vi "Power amplifier test.vi"() -> ()   [LabVIEW 2020]
uses:
  FunctionVi/Window/Control/Channel.ctl
  FunctionVi/Queue/Control/QueueState.ctl
  FunctionVi/Window/Control/Bit rate.ctl
  FunctionVi/Window/Control/HwType.ctl
  FunctionVi/Window/Control/Mode.ctl
  <vilib>/Utility/xml.llb/Read From XML File(string).vi
  <vilib>/Utility/file.llb/Write Delimited Spreadsheet (string).vi
  <vilib>/Utility/xml.llb/Read From XML File(array).vi
  <vilib>/Utility/xml.llb/Write to XML File(string).vi
  <userlib>/FTLDCPower/MPD.lvlib
  <userlib>/PCAN-Basic/PCANBasic.lvlib
  FunctionVi/Window/Win_PowerAmplifier_Transmit.vi
panel:
  out "x-y":u32
  out "Status":bool
  out "Company:":string
  out "Time:":string
  out "Channel:":T1 items=["PCAN_USBBUS1"=81, "PCAN_USBBUS2"=82, "PCAN_USBBUS3"=83, "PCAN_USBBUS4"=84]
  in  "PCAN Read error":string
  in  "source":string
  out "Status:":string
  out "Interface Information:":string
  in  "Max voltage:":dbl=30.0 min=5.0 format="%#.3gV"
  in  "BufferTime(s)":dbl=4.0 caption="Buffer:" format="%#.3gs"
  in  "ExecuteTime(s)":dbl=5.0 caption="Execute:" min=1.0 format="%#.3gs"
  in  "Step voltage:":dbl=0.1 format="%#.3gV"
  in  "Max voltage":dbl
  in  "At voltage":dbl
  in  "List record":i32(listbox)
  in  "Reset":bool
  in  "指示灯":bool
  in  "On/Off":bool
  in  "OCPEnable":bool
  in  "OCP:":dbl format="%#.3gA"
  in  "OVPEnable":bool
  in  "OVP:":dbl format="%#.3gV"
  in  "Current:":dbl format="%#.3gA"
  in  "Voltage:":dbl format="%#.3gV"
  in  "Transmit info":bool
  in  "Receive":i32(listbox)
  out "LastError":string
  in  "PCAN Config":bool
  out "Measure Voltage":dbl format="%#.3gV"
  out "Measure Power":dbl format="%#.3gW"
  out "Measure Current":dbl format="%#.3gA"
  in  "RS232 Config":bool
  # "Time"
  # "Output"
  # "Params Set"
  # "Measurement"
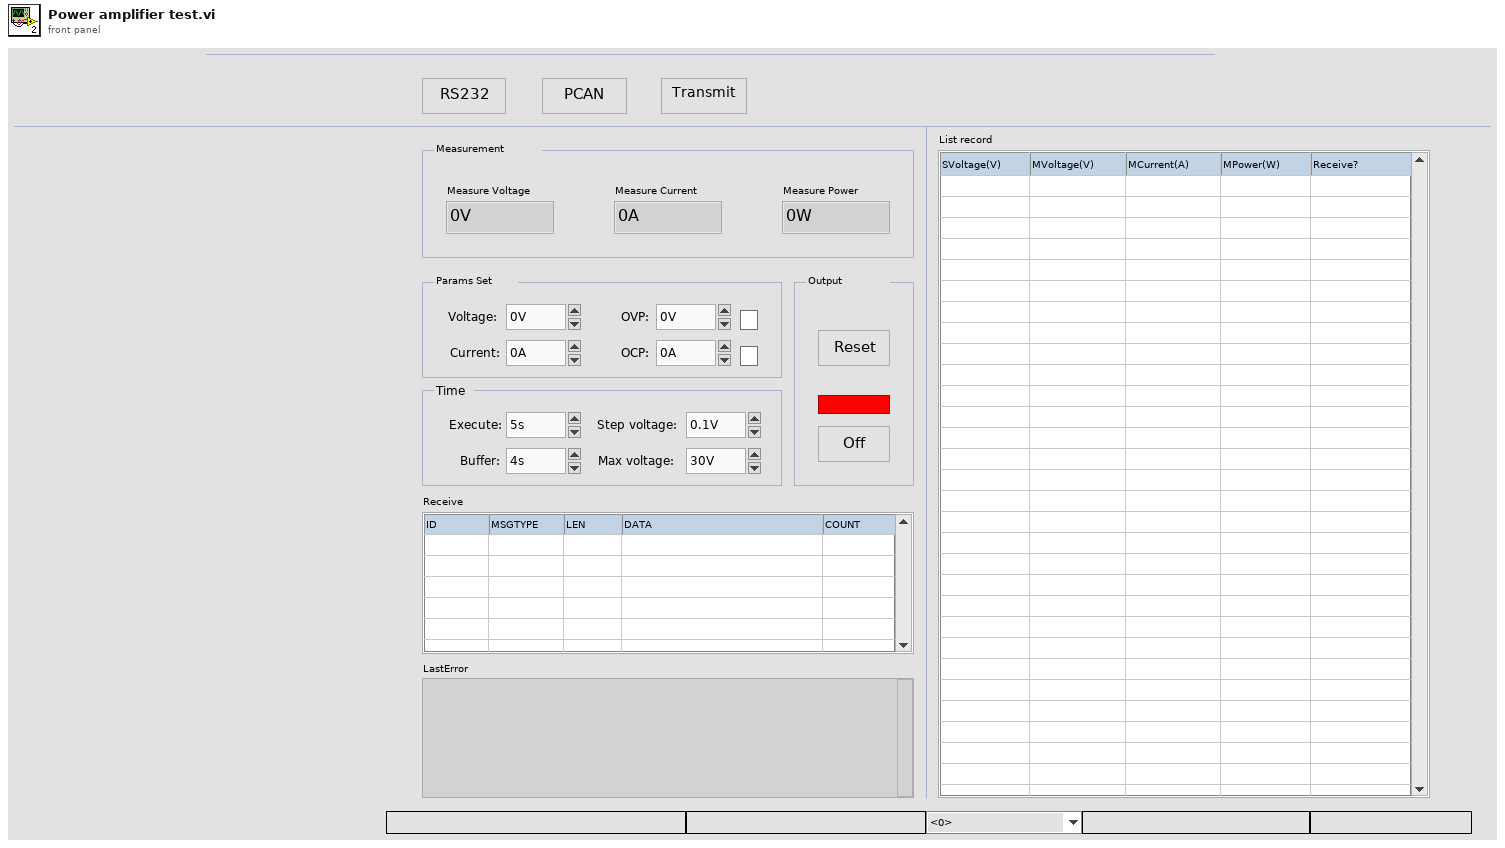
[diagram p1: front panel]
types:
  T1 = typedef "Channel.ctl" = u16
  T2 = typedef "QueueState.ctl" = enum16{"", "Create", "In", "Out", "Empty", "Close"}
  T3 = cluster{"ID":u32, "MSGTYPE":u8, "LEN":u8, "DATA[0]":u8, "DATA[1]":u8, "DATA[2]":u8, "DATA[3]":u8, "DATA[4]":u8, "DATA[5]":u8, "DATA[6]":u8, "DATA[7]":u8}
  T4 = cluster{"Baud Rate":u32, "Parity":u16, "Data Bits":u16, "Stop Bits":u16, "Flow Control":u16}
  T5 = typedef "Mode.ctl" = u8
  T6 = typedef "Bit rate.ctl" = u16
  T7 = typedef "HwType.ctl" = u8
  T8 = enum16{"VOLTage", "DEFault", "MINimum", "MAXimum"}
  T9 = enum16{"current", "DEFault", "MINimum", "MAXimum"}
  T10 = enum8{"Enabled", "Disabled", "Disabled and Grayed Out"}
  T11 = typedef "LVPoint32TypeDef.ctl" = cluster{"Horizontal":i32, "Vertical":i32}
  T12 = typedef "LVRowAndColumnTypeDef.ctl" = cluster{"Row":i32, "Column":i32}
  T13 = cluster{"ID":u32, "MSGTYPE":u8, "LEN":u8, "DATA[0]":u8, "DATA[1]":u8, "DATA[2]":u8, "DATA[3]":u8, "DATA[4]":u8, "DATA[5]":u8, "DATA[6]":u8, "DATA[7]":u8}[]
  T14 = cluster{"Time":u16, "MessageBuffer":cluster{"ID":u32, "MSGTYPE":u8, "LEN":u8, "DATA[0]":u8, "DATA[1]":u8, "DATA[2]":u8, "DATA[3]":u8, "DATA[4]":u8, "DATA[5]":u8, "DATA[6]":u8, "DATA[7]":u8}[]}[]
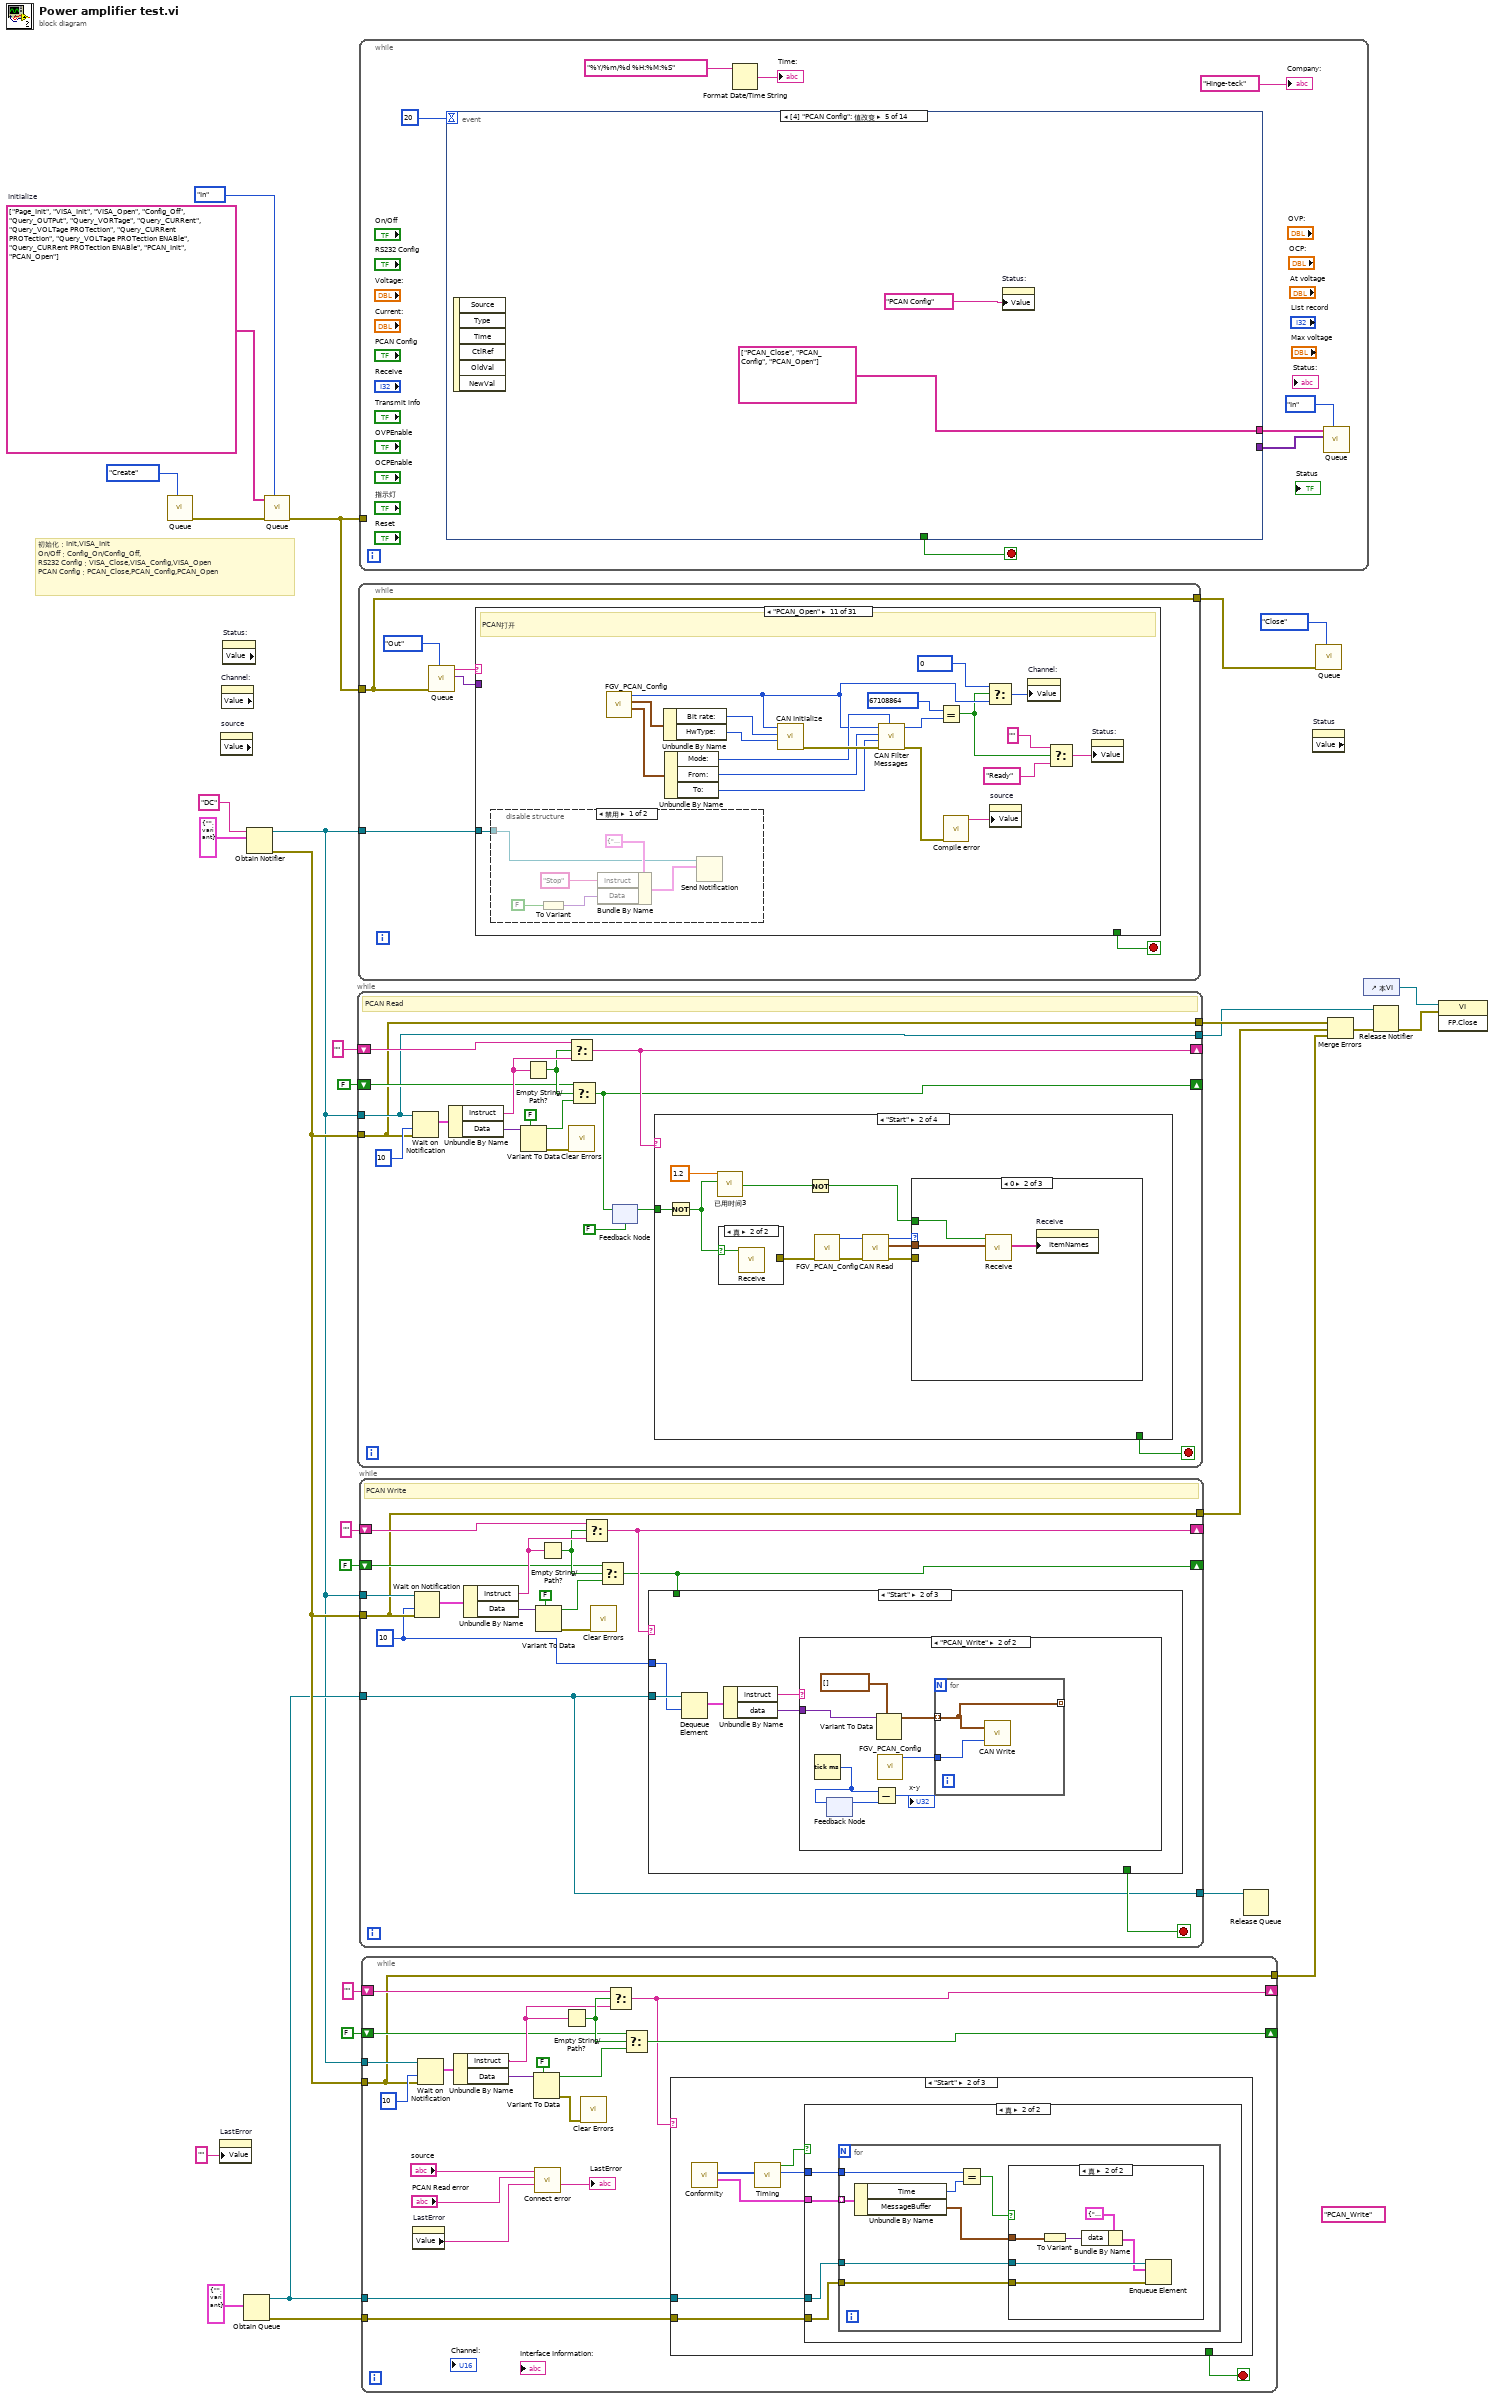
[diagram p0: block diagram]
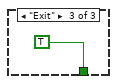
[diagram p5: hidden frame]
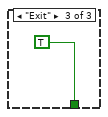
[diagram p8: hidden frame]
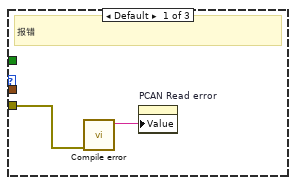
[diagram p10: hidden frame]
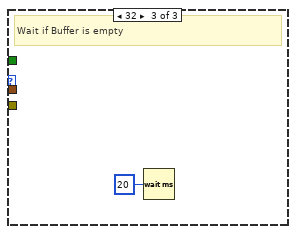
[diagram p11: hidden frame]
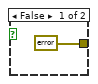
[diagram p12: hidden frame]
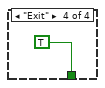
[diagram p14: hidden frame]
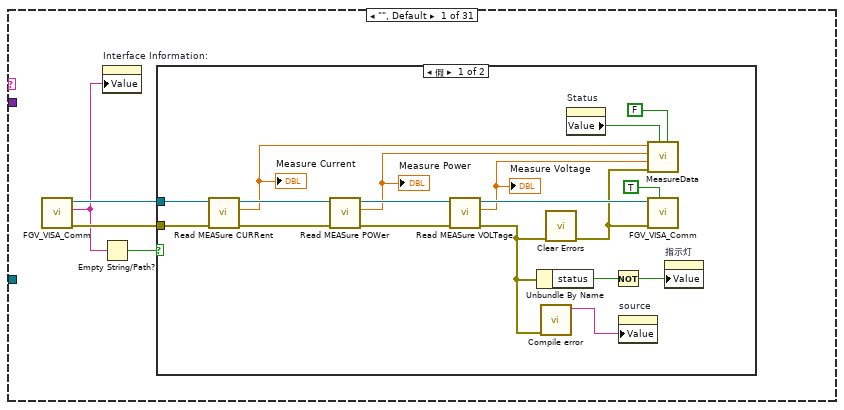
[diagram p15: hidden frame]
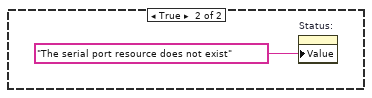
[diagram p16: hidden frame]
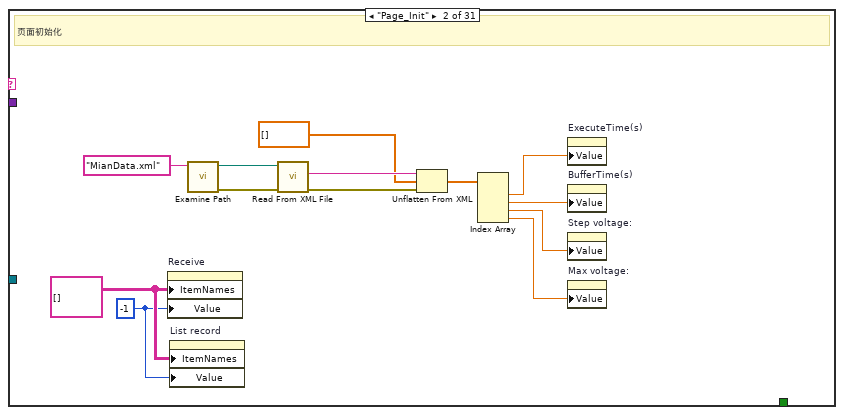
[diagram p17: hidden frame]
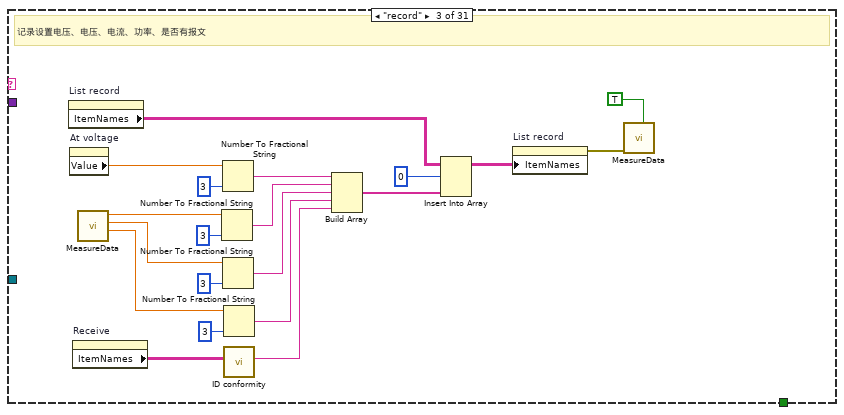
[diagram p18: hidden frame]
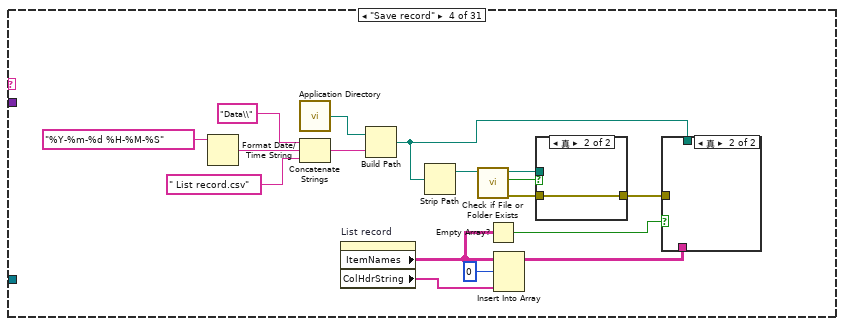
[diagram p19: hidden frame]
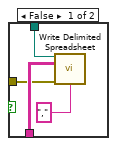
[diagram p20: hidden frame]
diagram:
  (unwired) "PCAN_Write"
  w25 = string[] ["Page_Init", "VISA_Init", "VISA_Open", "Config_Off", "Query_OUTPut", "Query_VORTage", "Query_CURRent", "Query_VOLTage PROTection", "Query_CURRent PROTection", "Query_VOLTage PROTection ENABle", "Query_CURRent PROTection ENABle", "PCAN_Init", "PCAN_Open"]  # Initialize
  # "初始化：Init,VISA_Init\nOn/Off：Config_On/Config_Off,\nRS232 Config：VISA_Close,VISA_Config,VISA_Open\nPCAN Config：PCAN_Close,PCAN_Config,PCAN_Open"
  n1 = call "Queue.vi"("State"=QueueState."Create") -> ("error out"=w28:errorcluster)  [unwired: 8 in, 2 out]
  n2 = property on="LastError" class="Str"("Value"="") -> ()  [unwired: 2 in, 2 out]
  n3 = property on="source" class="Str" props=["Value"]() -> ()  [unwired: 2 in, 3 out]
  n4 = property on="Channel:" class="Ring (严格)" props=["Value"]() -> ()  [unwired: 2 in, 3 out]
  n5 = property on="Status:" class="Str" props=["Value"]() -> ()  [unwired: 2 in, 3 out]
  n6 = Obtain Queue(element data type=cluster{"instruct":string, "data":variant} {"instruct"="", "data"=variant}) -> (queue out=w19:refnum<queue>, error out=w6:errorcluster)  [unwired: 4 in, 1 out]
  n7 = Obtain Notifier(name (unnamed)="DC" ("名称（未命名）"), notification data type=cluster{"Instruct":string, "Data":variant} {"Instruct"="", "Data"=variant}) -> (notifier out=w18:refnum<notifier>, error out=w20:errorcluster)  [unwired: 2 in, 1 out]
  n8 = call "Queue.vi"("State"=QueueState."In", "error in"=w28, "Instruct"=w25) -> ("error out"=w27:errorcluster)  [unwired: 6 in, 2 out]
  n9 = while {
    tunnel: w20 -> [w30]
    tunnel: w18 -> [w35]
    shift-right: [w37] -> _
    shift-left: "" ("Instruct") -> [w43]
    shift-right: [w33] -> _
    shift-left: FALSE -> [w38]
    tunnel: [w35] -> w12
    tunnel: [w30] -> w14
    stop <- w36 stop-if-true
    # "PCAN Read"
    n10 = Wait on Notification(notifier=w35, timeout in ms (-1)=10 ("超时毫秒(-1)"), error in (no error)=w30) -> (notification=w45:cluster{"Instruct":string, "Data":variant})  [unwired: 1 in, 3 out]
    n11 = Unbundle By Name(w45) -> ("Instruct"=w44:string, "Data"=w41:variant)
    n12 = Variant To Data(type=FALSE, Variant=w41) -> (data=w39:bool, error out=w34:errorcluster)  [unwired: 1 in]
    n13 = Empty String/Path?(string/path=w44) -> (empty?=w42:bool)
    n14 = Select(t=w43, s=w42, f=w44) -> (s? t:f=w37:string)
    n15 = call <vilib>:"Clear Errors.vi"("error in (no error)"=w34) -> ()  [unwired: 5 in, 2 out]
    n16 = Select(t=w38, s=w42, f=w39) -> (s? t:f=w33:bool)
    n17 = feedback-in #1(w33) -> ()
    n18 = feedback #1(FALSE) -> (w31:bool)
    n19 = case shown="\"Start\"" w37 {
      tunnel: [_ _ _ TRUE] -> w36
      tunnel: w31 -> [_ w57 _ _]
      frame "假", Default {
      }
      frame "Start" {
        n20 = Not(x=w57) -> (.not. x?=w55:bool)
        n21 = call "已用时间3"("Time Target (s)"=1.2, "Reset"=w55) -> ("Time has Elapsed"=w48:bool)  [unwired: 10 in, 7 out]
        n22 = case shown="真" w55 {
          selector: w55 -> [_ w65]
          tunnel: [errorcluster {"status"=FALSE, "code"=0, "source"=""} ("错误常量") _] -> w56
          frame False {
          }
          frame True {
            n23 = call "Receive.vi"("Clear?"=w65) -> ()  [unwired: 10 in, 1 out]
          }
        }
        n24 = Not(x=w48) -> (.not. x?=w47:bool)
        n25 = call "FGV_PCAN_Config.vi"("error in"=w56) -> ("error out"=w51:errorcluster, "Channel out"=w53:T1)  [unwired: 7 in, 2 out]
        n26 = call <userlib>:"CAN Read.vi"("error in (no error)"=w51, "Channel"=w53) -> ("error out"=w50:errorcluster, "MessageBuffer out"=w49:T3, "function return"=w52:u32)  [unwired: 6 in, 1 out]
        n27 = case shown="0" w52 {
          tunnel: w50 -> [w59 _ _]
          tunnel: w49 -> [_ w62 _]
          tunnel: w47 -> [_ w60 _]
          frame Default {
            # "报错"
            n28 = call "Compile error.vi"("错误输入"=w59) -> ("Error out"=w58:string)  [unwired: 10 in]
            n29 = property on="PCAN Read error" class="Str"("Value"=w58) -> ()  [unwired: 2 in, 2 out]
          }
          frame 0 {
            n30 = call "Receive.vi"("MessageBuffer"=w62, "Clear?"=w60) -> ("Receive"=w61:string[][])  [unwired: 9 in]
            n31 = property on="Receive" class="MCListbox (严格)"("ItemNames"=w61) -> ()  [unwired: 2 in, 2 out]
          }
          frame 32 {
            # "Wait if Buffer is empty"
            n32 = Wait (ms)(milliseconds to wait=u32 20 ("等待时间（毫秒）")) -> ()  [unwired: 1 out]
          }
        }
      }
      frame "Stop" {
      }
      frame "Exit" {
      }
    }
  }
  n33 = while {
    tunnel: w27 -> [w68]
    tunnel: w18 -> [w67]
    tunnel: [w68] -> w22
    stop <- w70 stop-if-true
    n34 = call "Queue.vi"("State"=QueueState."Out", "error in"=w68) -> ("Data Out"=w69:variant, "Instruct Out"=w71:string)  [unwired: 7 in, 1 out]
    n35 = case shown="\"PCAN_Open\"" w71 {
      tunnel: [_ _ _ _ _ _ _ _ _ _ _ _ _ _ _ _ _ _ _ _ _ _ _ _ _ _ _ _ _ _ TRUE] -> w70
      tunnel: w69 -> [_ _ _ _ _ _ _ _ _ _ _ _ _ _ w250 _ _ _ _ _ _ _ _ _ _ _ _ _ _ _ _]
      tunnel: w67 -> [_ _ _ _ _ _ _ _ _ _ w211 _ _ _ _ _ _ _ _ _ w296 w308 w328 _ _ _ _ _ _ _ w400]
      frame "", Default {
        n36 = call "FGV_VISA_Comm.vi"() -> ("error out"=w76:errorcluster, "Interface Information"=w73:string, "VISA resource name out"=w75:refnum<visa-resource-name>)  [unwired: 9 in]
        n37 = Empty String/Path?(string/path=w73) -> (empty?=w74:bool)
        n38 = property on="Interface Information:" class="Str"("Value"=w73) -> ()  [unwired: 2 in, 2 out]
        n39 = case shown="假" w74 {
          tunnel: w76 -> [w94 _]
          tunnel: w75 -> [w89 _]
          frame False {
            n40 = call <userlib>:"Read MEASure CURRent.vi"("error in (no error)"=w94, "VISA resource name"=w89) -> ("error out"=w93:errorcluster, "Measure Current"=w83:dbl, "VISA resource name out"=w90:refnum<visa-resource-name>)  [unwired: 7 in]
            "Measure Current" <- w83
            n41 = call <userlib>:"Read MEASure POWer.vi"("error in (no error)"=w93, "VISA resource name"=w90) -> ("error out"=w91:errorcluster, "Measure Power"=w82:dbl, "VISA resource name out"=w92:refnum<visa-resource-name>)  [unwired: 7 in]
            "Measure Power" <- w82
            n42 = call <userlib>:"Read MEASure VOLTage.vi"("error in (no error)"=w91, "VISA resource name"=w92) -> ("error out"=w80:errorcluster, "Measure VOLTage"=w81:dbl, "VISA resource name out"=w88:refnum<visa-resource-name>)  [unwired: 7 in]
            "Measure Voltage" <- w81
            n43 = Unbundle By Name(w80) -> ("status"=w86:bool)
            n44 = call "Compile error.vi"("错误输入"=w80) -> ("Error out"=w79:string)  [unwired: 10 in]
            n45 = call <vilib>:"Clear Errors.vi"("error in (no error)"=w80) -> ("error out"=w84:errorcluster)  [unwired: 5 in, 1 out]
            n46 = property on="Status" class="Bool (严格)"() -> ("Value"=w78:bool)  [unwired: 2 in, 2 out]
            n47 = Not(x=w86) -> (.not. x?=w85:bool)
            n48 = property on="source" class="Str"("Value"=w79) -> ()  [unwired: 2 in, 2 out]
            n49 = call "MeasureData.vi"("Reset?"=FALSE, "Write?"=w78, "error in"=w84, "Measure Voltage"=w81, "Measure Power"=w82, "Measure Current"=w83) -> ()  [unwired: 2 in, 4 out]
            n50 = call "FGV_VISA_Comm.vi"("Write?"=TRUE, "error in"=w84, "VISA resource name"=w88) -> ()  [unwired: 6 in, 3 out]
            n51 = property on="指示灯" class="Bool (严格)"("Value"=w85) -> ()  [unwired: 2 in, 2 out]
          }
          frame True {
            n52 = property on="Status:" class="Str"("Value"="The serial port resource does not exist") -> ()  [unwired: 2 in, 2 out]
          }
        }
      }
      frame "Page_Init" {
        w107 = -1 ("Receive")
        w108 = string[][] [] ("项名")
        # "页面初始化"
        n53 = property on="Receive" class="MCListbox (严格)"("ItemNames"=w108, "Value"=w107) -> ()  [unwired: 2 in, 2 out]
        n54 = property on="List record" class="MCListbox (严格)"("ItemNames"=w108, "Value"=w107) -> ()  [unwired: 2 in, 2 out]
        n55 = call "Examine Path.vi"("Filename"="MianData.xml") -> ("error out"=w104:errorcluster, "Path"=w105:path)  [unwired: 9 in]
        n56 = call-poly <vilib>:"Read From XML File.vi"("error in (no error)"=w104, "XML File Path"=w105) -> ("error out"=w102:errorcluster, "XML Elements"=w103:string)  [unwired: 7 in, 1 out]
        n57 = Unflatten From XML(xml string=w103, type=dbl[] [], error in (no error)=w102) -> (value=w100:dbl[])  [unwired: 1 out]
        n58 = Index Array(array=w100) -> (element #1=w99:dbl, element #2=w98:dbl, element #3=w97:dbl, element #4=w96:dbl)  [unwired: 4 in]
        n59 = property on="ExecuteTime(s)" class="DigNum (严格)"("Value"=w99) -> ()  [unwired: 2 in, 2 out]
        n60 = property on="BufferTime(s)" class="DigNum (严格)"("Value"=w98) -> ()  [unwired: 2 in, 2 out]
        n61 = property on="Step voltage:" class="DigNum (严格)"("Value"=w97) -> ()  [unwired: 2 in, 2 out]
        n62 = property on="Max voltage:" class="DigNum (严格)"("Value"=w96) -> ()  [unwired: 2 in, 2 out]
      }
      frame "record" {
        # "记录设置电压、电压、电流、功率、是否有报文"
        n63 = property on="List record" class="MCListbox (严格)"() -> ("ItemNames"=w117:string[][])  [unwired: 2 in, 2 out]
        n64 = property on="At voltage" class="DigNum (严格)"() -> ("Value"=w128:dbl)  [unwired: 2 in, 2 out]
        n65 = property on="Receive" class="MCListbox (严格)"() -> ("ItemNames"=w123:string[][])  [unwired: 2 in, 2 out]
        n66 = call "MeasureData.vi"() -> ("PowerAverage(..10)"=w111:dbl, "CurrentAverage(..10)"=w112:dbl, "VoltageAverage(..10)"=w113:dbl)  [unwired: 8 in, 1 out]
        n67 = Number To Fractional String(number=w113, precision (6)=i16 3 ("精度(6)")) -> (F-format string=w121:string)  [unwired: 2 in]
        n68 = Number To Fractional String(number=w128, precision (6)=i16 3 ("精度(6)")) -> (F-format string=w122:string)  [unwired: 2 in]
        n69 = Number To Fractional String(number=w112, precision (6)=i16 3 ("精度(6)")) -> (F-format string=w120:string)  [unwired: 2 in]
        n70 = Number To Fractional String(number=w111, precision (6)=i16 3 ("精度(6)")) -> (F-format string=w119:string)  [unwired: 2 in]
        n71 = call "ID conformity.vi"("项名"=w123) -> ("ID conformity"=w118:string)  [unwired: 10 in]
        n72 = Build Array(w122, w121, w120, w119, w118) -> (w116:string[])
        n73 = Insert Into Array(array=w117, index (row)=0 ("索引 (行)"), new element=w116) -> (w114:string[][])  [unwired: 1 in]
        n74 = property on="List record" class="MCListbox (严格)"("ItemNames"=w114) -> (error out=w110:errorcluster)  [unwired: 2 in, 1 out]
        n75 = call "MeasureData.vi"("Reset?"=TRUE, "error in"=w110) -> ()  [unwired: 6 in, 4 out]
      }
      frame "Save record" {
        n76 = Format Date/Time String(time format string (%c)="%Y-%m-%d %H-%M-%S" ("时间格式字符串(%c)")) -> (date/time string=w142:string)  [unwired: 2 in]
        n77 = call <vilib>:"Application Directory.vi"() -> ("Application Directory"=w145:path)
        n78 = Concatenate Strings("Data\\" ("字符串"), w142, " List record.csv" ("字符串")) -> (w140:string)
        n79 = property on="List record" class="MCListbox (严格)"() -> ("ItemNames"=w130:string[][], "ColHdrString"=w139:string[])  [unwired: 2 in, 2 out]
        n80 = Build Path(base path=w145, name or relative path=w140) -> (appended path=w131:path)
        n81 = Strip Path(path=w131) -> (stripped path=w136:path)  [unwired: 1 out]
        n82 = call <vilib>:"Check if File or Folder Exists.vi"("path"=w136) -> ("error out"=w133:errorcluster, "file or folder exists?"=w135:bool, "dup path"=w134:path)  [unwired: 8 in]
        n83 = Empty Array?(array=w130) -> (empty?=w129:bool)
        n84 = Insert Into Array(array=w130, index (row)=0 ("索引 (行)"), new element=w139) -> (w137:string[][])  [unwired: 1 in]
        n85 = case shown="真" w135 {
          tunnel: w134 -> [w152 _]
          tunnel: w133 -> [w151 w153]
          tunnel: [w150 w153] -> w132
          frame False {
            n86 = Create Folder(path (use dialog)=w152, error in=w151) -> (error out=w150:errorcluster)  [unwired: 1 in, 2 out]
          }
          frame True {
          }
        }
        n87 = case shown="真" w129 {
          tunnel: w137 -> [w148 _]
          tunnel: w132 -> [w147 _]
          tunnel: w131 -> [w146 _]
          frame False {
            n88 = call-poly <vilib>:"Write Delimited Spreadsheet.vi"("file path (dialog if empty)"=w146, "2D data"=w148, "error in (no error)"=w147, "delimiter (\\t)"="," ("delimiter (\\t)")) -> ()  [unwired: 10 in, 2 out]
          }
          frame True {
          }
        }
      }
      frame "VISA_Init" {
        # "VISA初始化"
        n89 = call "Examine Path.vi"("Filename"="RS232Data.xml") -> ("error out"=w161:errorcluster, "Path"=w162:path)  [unwired: 9 in]
        n90 = call-poly <vilib>:"Read From XML File.vi"("error in (no error)"=w161, "XML File Path"=w162) -> ("XML Elements"=w160:string[])  [unwired: 7 in, 2 out]
        n91 = Index Array(array=w160) -> (element #1=w159:string, element #2=w156:string)  [unwired: 2 in]
        n92 = Unflatten From XML(xml string=w156, type=T4 {"Baud Rate"=9600, "Parity"=0, "Data Bits"=8, "Stop Bits"=10, "Flow Control"=0} ("Serial Configuration")) -> (value=w154:T4)  [unwired: 1 in, 1 out]
        n93 = Unflatten From XML(xml string=w159, type=refnum<visa-resource-name> refnum ("CommName:")) -> (value=w157:refnum<visa-resource-name>)  [unwired: 1 in, 1 out]
        n94 = call "FGV_VISA_Config.vi"("Write?"=TRUE, "Serial Configuration"=w154, "CommName"=w157) -> ()  [unwired: 6 in, 3 out]
      }
      frame "VISA_Config" {
        # "VISA配置参数"
        n95 = call-by-ref "?"() -> ("Yes out"=w165:bool)  [unwired: 10 in, 5 out]
        n96 = case shown="真" w165 {
          frame False {
          }
          frame True {
            n97 = vi-ref "Win_RS232_Config.vi"() -> (w167:refnum<vi>)
            n98 = invoke class="VI" method="Default Vals.Make Curr Default"(reference=w167) -> (reference out=w166:refnum<vi>)  [unwired: 2 in, 2 out]
            n99 = Close Reference(reference=w166) -> ()  [unwired: 1 in, 1 out]
          }
        }
      }
      frame "VISA_Open" {
        # "VISA连接"
        n100 = call "FGV_VISA_Config.vi"() -> ("error out"=w182:errorcluster, "Serial Configuration Out"=w180:T4, "CommNameOut"=w181:refnum<visa-resource-name>)  [unwired: 9 in]
        n101 = call <userlib>:"Close.vi"("error in (no error)"=w182, "VISA resource name"=w181) -> ("error out"=w179:errorcluster)  [unwired: 9 in]
        n102 = call <vilib>:"Clear Errors.vi"("error in (no error)"=w179) -> ("error out"=w178:errorcluster)  [unwired: 5 in, 1 out]
        n103 = call <userlib>:"Initialize.vi"("VISA resource name"=w181, "Serial Configuration"=w180, "error in (no error)"=w178) -> ("VISA resource name out"=w170:refnum<visa-resource-name>, "error out"=w176:errorcluster)  [unwired: 6 in]
        n104 = Unbundle By Name(w176) -> ("code"=w175:i32)
        n105 = call "Compile error.vi"("错误输入"=w176) -> ("Error out"=w168:string)  [unwired: 10 in]
        n106 = property on="source" class="Str"("Value"=w168) -> ()  [unwired: 2 in, 2 out]
        n107 = Equal?(x=w175, y=-1073807343) -> (x = y?=w172:bool)
        n108 = Select(t=refnum<visa-resource-name> refnum ("VISA resource name"), s=w172, f=w170) -> (s? t:f=w169:refnum<visa-resource-name>)
        n109 = case shown="假" w172 {
          frame False {
          }
          frame True {
            n110 = call "Queue.vi"("State"=QueueState."Empty") -> ()  [unwired: 8 in, 3 out]
          }
        }
        n111 = call "FGV_VISA_Comm.vi"("Write?"=TRUE, "error in"=w176, "VISA resource name"=w169) -> ("error out"=w177:errorcluster)  [unwired: 6 in, 2 out]
        n112 = call <vilib>:"Clear Errors.vi"("error in (no error)"=w177) -> ()  [unwired: 5 in, 2 out]
      }
      frame "VISA_Close" {
        # "VISA关闭连接"
        n113 = call "FGV_VISA_Comm.vi"() -> ("error out"=w185:errorcluster, "VISA resource name out"=w186:refnum<visa-resource-name>)  [unwired: 9 in, 1 out]
        n114 = call <userlib>:"Close.vi"("error in (no error)"=w185, "VISA resource name"=w186) -> ("error out"=w184:errorcluster)  [unwired: 9 in]
        n115 = call <vilib>:"Clear Errors.vi"("error in (no error)"=w184) -> ()  [unwired: 5 in, 2 out]
      }
      frame "PCAN_Init" {
        w194 = T1 81 items=["PCAN_USBBUS1"=81, "PCAN_USBBUS2"=82, "PCAN_USBBUS3"=83, "PCAN_USBBUS4"=84] ("Channel:")
        # "PCAN读取配置"
        n116 = call "Examine Path.vi"("Filename"="TransmitData.xml") -> ("error out"=w204:errorcluster, "Path"=w205:path)  [unwired: 9 in]
        n117 = call "Examine Path.vi"("Filename"="PCANData.xml") -> ("error out"=w197:errorcluster, "Path"=w198:path)  [unwired: 9 in]
        n118 = call-poly <vilib>:"Read From XML File.vi"("error in (no error)"=w204, "XML File Path"=w205) -> ("XML Elements"=w203:string)  [unwired: 7 in, 2 out]
        n119 = call-poly <vilib>:"Read From XML File.vi"("error in (no error)"=w197, "XML File Path"=w198) -> ("XML Elements"=w196:string[])  [unwired: 7 in, 2 out]
        n120 = Index Array(array=w196) -> (element #1=w195:string, element #2=w192:string, element #3=w189:string)  [unwired: 3 in]
        n121 = Unflatten From XML(xml string=w203, type=string[][] []) -> (value=w201:string[][])  [unwired: 1 in, 1 out]
        n122 = Unflatten From XML(xml string=w195, type=w194) -> (value=w193:T1)  [unwired: 1 in, 1 out]
        n123 = call "FGV_PowerAmplifier_Transmit.vi"("Write?"=TRUE, "Transmit"=w201) -> ()  [unwired: 8 in, 2 out]
        n124 = Unflatten From XML(xml string=w192, type=cluster{"Bit rate:":T6, "HwType: ":T7} {"Bit rate:"=28, "HwType: "=1} ("Initialize")) -> (value=w190:cluster{"Bit rate:":T6, "HwType: ":T7})  [unwired: 1 in, 1 out]
        n125 = Unflatten From XML(xml string=w189, type=cluster{"Mode: ":T5, "From:":u32, "To:":u32} {"Mode: "=0, "From:"=0, "To:"=0} ("FilterMessages")) -> (value=w187:cluster{"Mode: ":T5, "From:":u32, "To:":u32})  [unwired: 1 in, 1 out]
        n126 = call "FGV_PCAN_Config.vi"("Write?"=TRUE, "FilterMessages"=w187, "Initialize"=w190, "Channel"=w193) -> ()  [unwired: 4 in, 4 out]
      }
      frame "PCAN_Config" {
        # "PCAN配置"
        n127 = call-by-ref "?"() -> ("Yes out"=w208:bool)  [unwired: 9 in, 6 out]
        n128 = case shown="真" w208 {
          frame False {
          }
          frame True {
            n129 = vi-ref "Win_PCAN_Config.vi"() -> (w210:refnum<vi>)
            n130 = invoke class="VI" method="Default Vals.Make Curr Default"(reference=w210) -> (reference out=w209:refnum<vi>)  [unwired: 2 in, 2 out]
            n131 = Close Reference(reference=w209) -> ()  [unwired: 1 in, 1 out]
          }
        }
      }
      frame "PCAN_Open" {
        w217 = T1 0 items=["PCAN_USBBUS1"=81, "PCAN_USBBUS2"=82, "PCAN_USBBUS3"=83, "PCAN_USBBUS4"=84] ("t")
        # "PCAN打开"
        n132 = disable-structure shown="禁用" {
          disable-tunnel: w211 -> [w231 _]
          frame Disabled {
            n133 = To Variant(anything=FALSE) -> (Variant=w233:variant)
            n134 = Bundle By Name(cluster=cluster{"Instruct":string, "Data":variant} {"Instruct"="", "Data"=variant}, "Instruct"="Stop", "Data"=w233) -> (w236:cluster{"Instruct":string, "Data":variant})
            n135 = Send Notification(notification=w236, notifier=w231) -> ()  [unwired: 1 in, 2 out]
          }
          frame Enabled {
          }
        }
        n136 = call "FGV_PCAN_Config.vi"() -> ("FilterMessages out"=w229:cluster{"Mode: ":T5, "From:":u32, "To:":u32}, "Initialize out"=w230:cluster{"Bit rate:":T6, "HwType: ":T7}, "Channel out"=w218:T1)  [unwired: 8 in, 1 out]
        n137 = Unbundle By Name(w230) -> ("Bit rate:"=w228:T6, "HwType:"=w227:T7)
        n138 = Unbundle By Name(w229) -> ("Mode:"=w225:T5, "From:"=w224:u32, "To:"=w223:u32)
        n139 = call <userlib>:"CAN Initialize.vi"("HwType"=w227, "Btr0Btr1"=w228, "Channel"=w218) -> ("错误输出"=w226:errorcluster)  [unwired: 7 in, 1 out]
        n140 = call <userlib>:"CAN Filter Messages.vi"("Mode"=w225, "error in (no error)"=w226, "ToID"=w223, "FromID"=w224, "Channel"=w218) -> ("error out"=w222:errorcluster, "function return"=w220:u32)  [unwired: 5 in]
        n141 = Equal?(x=u32 67108864, y=w220) -> (x = y?=w215:bool)
        n142 = call "Compile error.vi"("错误输入"=w222) -> ("Error out"=w221:string)  [unwired: 10 in]
        n143 = Select(t=w217, s=w215, f=w218) -> (s? t:f=w216:T1)
        n144 = property on="source" class="Str"("Value"=w221) -> ()  [unwired: 2 in, 2 out]
        n145 = property on="Channel:" class="Ring (严格)"("Value"=w216) -> ()  [unwired: 2 in, 2 out]
        n146 = Select(t="", s=w215, f="Ready") -> (s? t:f=w212:string)
        n147 = property on="Status:" class="Str"("Value"=w212) -> ()  [unwired: 2 in, 2 out]
      }
      frame "PCAN_Close" {
        # "PCAN关闭"
        n148 = call "FGV_PCAN_Config.vi"() -> ("Channel out"=w237:T1)  [unwired: 8 in, 3 out]
        n149 = call <userlib>:"CAN Uninitialize.vi"("Channel"=w237) -> ()  [unwired: 10 in, 1 out]
      }
      frame "Transmit_info" {
        # "报文"
        n150 = call-by-ref "?"() -> ("Yes out"=w238:bool)  [unwired: 12 in, 3 out]
        n151 = case shown="真" w238 {
          frame False {
          }
          frame True {
            n152 = vi-ref "Win_PCAN_Config.vi"() -> (w240:refnum<vi>)
            n153 = invoke class="VI" method="Default Vals.Make Curr Default"(reference=w240) -> (reference out=w239:refnum<vi>)  [unwired: 2 in, 2 out]
            n154 = Close Reference(reference=w239) -> ()  [unwired: 1 in, 1 out]
          }
        }
      }
      frame "Config_VOLTage" {
        # "设置输出电压"
        n155 = call "FGV_VISA_Comm.vi"() -> ("error out"=w244:errorcluster, "VISA resource name out"=w246:refnum<visa-resource-name>)  [unwired: 9 in, 1 out]
        n156 = property on="Voltage:" class="DigNum (严格)"() -> ("Value"=w241:dbl)  [unwired: 2 in, 2 out]
        n157 = call <userlib>:"Configure VOLTage LEVel.vi"("VOLTage  Value(V)"=w241, "error in (no error)"=w244, "VOLTage Tab"=T8."VOLTage", "VISA resource name"=w246) -> ("error out"=w243:errorcluster, "VISA resource name out"=w245:refnum<visa-resource-name>)  [unwired: 6 in]
        n158 = call "FGV_VISA_Comm.vi"("Write?"=TRUE, "error in"=w243, "VISA resource name"=w245) -> ()  [unwired: 6 in, 3 out]
      }
      frame "Config_VOLTage1" {
        # "设置输出电压"
        n159 = Variant To Data(type=0.0 ("x+y"), Variant=w250) -> (data=w248:dbl)  [unwired: 1 in, 1 out]
        n160 = call "FGV_VISA_Comm.vi"() -> ("error out"=w253:errorcluster, "VISA resource name out"=w255:refnum<visa-resource-name>)  [unwired: 9 in, 1 out]
        n161 = call <userlib>:"Configure VOLTage LEVel.vi"("VOLTage  Value(V)"=w248, "error in (no error)"=w253, "VOLTage Tab"=T8."VOLTage", "VISA resource name"=w255) -> ("error out"=w252:errorcluster, "VISA resource name out"=w254:refnum<visa-resource-name>)  [unwired: 6 in]
        n162 = call "FGV_VISA_Comm.vi"("Write?"=TRUE, "error in"=w252, "VISA resource name"=w254) -> ()  [unwired: 6 in, 3 out]
      }
      frame "Config_CURRent" {
        # "设置输出电流"
        n163 = call "FGV_VISA_Comm.vi"() -> ("error out"=w259:errorcluster, "VISA resource name out"=w260:refnum<visa-resource-name>)  [unwired: 9 in, 1 out]
        n164 = property on="Current:" class="DigNum (严格)"() -> ("Value"=w257:dbl)  [unwired: 2 in, 2 out]
        n165 = call <userlib>:"Configure CURRent LEVel.vi"("Current  Value(A)"=w257, "error in (no error)"=w259, "Current Tab"=T9."current", "VISA resource name"=w260) -> ("error out"=w261:errorcluster, "VISA resource name out"=w262:refnum<visa-resource-name>)  [unwired: 6 in]
        n166 = call "FGV_VISA_Comm.vi"("Write?"=TRUE, "error in"=w261, "VISA resource name"=w262) -> ()  [unwired: 6 in, 3 out]
      }
      frame "Config_VOLTage PROTection" {
        # "设置输出电压保护阈值"
        n167 = call "FGV_VISA_Comm.vi"() -> ("error out"=w267:errorcluster, "VISA resource name out"=w266:refnum<visa-resource-name>)  [unwired: 9 in, 1 out]
        n168 = property on="OVP:" class="DigNum (严格)"() -> ("Value"=w264:dbl)  [unwired: 2 in, 2 out]
        n169 = call <userlib>:"Configure VOLTage PROTection LEVel.vi"("VISA resource name"=w266, "VOLTage Tab"=T8."VOLTage", "VOLTage Protection Value(V)"=w264, "error in (no error)"=w267) -> ("VISA resource name out"=w269:refnum<visa-resource-name>, "error out"=w268:errorcluster)  [unwired: 4 in]
        n170 = call "FGV_VISA_Comm.vi"("Write?"=TRUE, "error in"=w268, "VISA resource name"=w269) -> ()  [unwired: 6 in, 3 out]
      }
      frame "Config_CURRent PROTection" {
        # "设置输出电流保护阈值"
        n171 = call "FGV_VISA_Comm.vi"() -> ("error out"=w273:errorcluster, "VISA resource name out"=w274:refnum<visa-resource-name>)  [unwired: 9 in, 1 out]
        n172 = property on="OCP:" class="DigNum (严格)"() -> ("Value"=w271:dbl)  [unwired: 2 in, 2 out]
        n173 = call <userlib>:"Configure CURRent PROTection LEVel.vi"("VISA resource name"=w274, "Current Tab"=T9."current", "Current Protection Value(A)"=w271, "error in (no error)"=w273) -> ("VISA resource name out"=w276:refnum<visa-resource-name>, "error out"=w275:errorcluster)  [unwired: 4 in]
        n174 = call "FGV_VISA_Comm.vi"("Write?"=TRUE, "error in"=w275, "VISA resource name"=w276) -> ()  [unwired: 6 in, 3 out]
      }
      frame "Config_VOLTage PROTection ENABle" {
        # "禁止或使能当前输出电压保护电路"
        n175 = call "FGV_VISA_Comm.vi"() -> ("error out"=w280:errorcluster, "VISA resource name out"=w281:refnum<visa-resource-name>)  [unwired: 9 in, 1 out]
        n176 = property on="OVPEnable" class="Bool (严格)"() -> ("Value"=w278:bool)  [unwired: 2 in, 2 out]
        n177 = call <userlib>:"Configure VOLTage PROTection ENABle.vi"("error in (no error)"=w280, "Enable VOLTage protection (T: Enable)"=w278, "VISA resource name"=w281) -> ("error out"=w279:errorcluster, "VISA resource name out"=w282:refnum<visa-resource-name>)  [unwired: 7 in]
        n178 = call "FGV_VISA_Comm.vi"("Write?"=TRUE, "error in"=w279, "VISA resource name"=w282) -> ()  [unwired: 6 in, 3 out]
      }
      frame "Config_CURRent PROTection ENABle" {
        # "禁止或使能当前输出电压保护电路"
        n179 = call "FGV_VISA_Comm.vi"() -> ("error out"=w285:errorcluster, "VISA resource name out"=w286:refnum<visa-resource-name>)  [unwired: 9 in, 1 out]
        n180 = property on="OCPEnable" class="Bool (严格)"() -> ("Value"=w284:bool)  [unwired: 2 in, 2 out]
        n181 = call <userlib>:"Configure CURRent PROTection ENABle.vi"("error in (no error)"=w285, "Enable Current protection (T: Enable)"=w284, "VISA resource name"=w286) -> ("error out"=w287:errorcluster, "VISA resource name out"=w288:refnum<visa-resource-name>)  [unwired: 7 in]
        n182 = call "FGV_VISA_Comm.vi"("Write?"=TRUE, "error in"=w287, "VISA resource name"=w288) -> ()  [unwired: 6 in, 3 out]
      }
      frame "Config_On" {
        # "VISA打开通道"
        n183 = To Variant(anything=TRUE) -> (Variant=w291:variant)
        n184 = call "FGV_VISA_Comm.vi"() -> ("error out"=w301:errorcluster, "VISA resource name out"=w302:refnum<visa-resource-name>)  [unwired: 9 in, 1 out]
        n185 = Bundle By Name(cluster=cluster{"Instruct":string, "Data":variant} {"Instruct"="", "Data"=variant} ("通知"), "Instruct"="Start", "Data"=w291) -> (w294:cluster{"Instruct":string, "Data":variant})
        n186 = call <userlib>:"Configure OUTPut ENABle.vi"("error in (no error)"=w301, "Enable OUTPut (T: Enable)"=TRUE, "VISA resource name"=w302) -> ("error out"=w297:errorcluster, "VISA resource name out"=w299:refnum<visa-resource-name>)  [unwired: 7 in]
        n187 = Send Notification(notification=w294, notifier=w296) -> ()  [unwired: 1 in, 2 out]
        n188 = call "FGV_VISA_Comm.vi"("Write?"=TRUE, "error in"=w297, "VISA resource name"=w299) -> ()  [unwired: 6 in, 3 out]
        n189 = property on="Status" class="Bool (严格)"("Value"=TRUE ("Status")) -> ()  [unwired: 2 in, 2 out]
      }
      frame "Config_Off" {
        # "VISA关闭通道"
        n190 = To Variant(anything=FALSE) -> (Variant=w309:variant)
        n191 = Bundle By Name(cluster=cluster{"Instruct":string, "Data":variant} {"Instruct"="", "Data"=variant}, "Instruct"="Stop", "Data"=w309) -> (w312:cluster{"Instruct":string, "Data":variant})
        n192 = call "FGV_VISA_Comm.vi"() -> ("error out"=w316:errorcluster, "VISA resource name out"=w317:refnum<visa-resource-name>)  [unwired: 9 in, 1 out]
        n193 = Send Notification(notification=w312, notifier=w308) -> ()  [unwired: 1 in, 2 out]
        n194 = call <userlib>:"Configure OUTPut ENABle.vi"("error in (no error)"=w316, "Enable OUTPut (T: Enable)"=FALSE, "VISA resource name"=w317) -> ("error out"=w305:errorcluster, "VISA resource name out"=w314:refnum<visa-resource-name>)  [unwired: 7 in]
        n195 = call "Compile error.vi"("错误输入"=w305) -> ("Error out"=w304:string)  [unwired: 10 in]
        n196 = call <vilib>:"Clear Errors.vi"("error in (no error)"=w305) -> ("error out"=w306:errorcluster)  [unwired: 5 in, 1 out]
        n197 = call "FGV_VISA_Comm.vi"("Write?"=TRUE, "error in"=w306, "VISA resource name"=w314) -> ()  [unwired: 6 in, 3 out]
        n198 = property on="Status" class="Bool (严格)"("Value"=FALSE ("Status")) -> ()  [unwired: 2 in, 2 out]
        n199 = property on="source" class="Str"("Value"=w304) -> ()  [unwired: 2 in, 2 out]
      }
      frame "Config_Reset" {
        # "VISA关闭通道、清除保护电路"
        n200 = call "FGV_VISA_Comm.vi"() -> ("error out"=w335:errorcluster, "VISA resource name out"=w336:refnum<visa-resource-name>)  [unwired: 9 in, 1 out]
        n201 = To Variant(anything=FALSE) -> (Variant=w329:variant)
        n202 = call <userlib>:"Configure OUTPut ENABle.vi"("error in (no error)"=w335, "Enable OUTPut (T: Enable)"=FALSE, "VISA resource name"=w336) -> ("error out"=w325:errorcluster, "VISA resource name out"=w326:refnum<visa-resource-name>)  [unwired: 7 in]
        n203 = Bundle By Name(cluster=cluster{"Instruct":string, "Data":variant} {"Instruct"="", "Data"=variant}, "Instruct"="Stop", "Data"=w329) -> (w332:cluster{"Instruct":string, "Data":variant})
        n204 = call <userlib>:"Configure VOLTage PROTection CLEar.vi"("error in (no error)"=w325, "VISA resource name"=w326) -> ("error out"=w323:errorcluster, "VISA resource name out"=w324:refnum<visa-resource-name>)  [unwired: 8 in]
        n205 = Send Notification(notification=w332, notifier=w328) -> ()  [unwired: 1 in, 2 out]
        n206 = call <userlib>:"Configure CURRent PROTection CLEar.vi"("error in (no error)"=w323, "VISA resource name"=w324) -> ("error out"=w322:errorcluster, "VISA resource name out"=w321:refnum<visa-resource-name>)  [unwired: 8 in]
        n207 = call <userlib>:"Read OUTPut ENABle.vi"("error in (no error)"=w322, "等待时间（毫秒）"=u32 50, "VISA resource name"=w321) -> ("error out"=w318:errorcluster, "VISA resource name out"=w319:refnum<visa-resource-name>)  [unwired: 6 in, 1 out]
        n208 = call "FGV_VISA_Comm.vi"("Write?"=TRUE, "error in"=w318, "VISA resource name"=w319) -> ()  [unwired: 6 in, 3 out]
      }
      frame "Query_VORTage" {
        # "查询当前输出电压值"
        n209 = call "FGV_VISA_Comm.vi"() -> ("error out"=w347:errorcluster, "VISA resource name out"=w348:refnum<visa-resource-name>)  [unwired: 9 in, 1 out]
        n210 = call <userlib>:"Read VOLTage.vi"("error in (no error)"=w347, "等待时间（毫秒）"=u32 50, "VOLTage Tab"=T8."VOLTage", "VISA resource name"=w348) -> ("error out"=w342:errorcluster, "VOLTage  Value"=w345:dbl, "VISA resource name out"=w343:refnum<visa-resource-name>)  [unwired: 5 in]
        n211 = property on="Voltage:" class="DigNum (严格)"("Value"=w345) -> ()  [unwired: 2 in, 2 out]
        n212 = call <userlib>:"Read VOLTage.vi"("error in (no error)"=w342, "等待时间（毫秒）"=u32 50, "VOLTage Tab"=T8."MAXimum", "VISA resource name"=w343) -> ("error out"=w340:errorcluster, "VOLTage  Value"=w337:dbl, "VISA resource name out"=w341:refnum<visa-resource-name>)  [unwired: 5 in]
        n213 = property on="Max voltage" class="DigNum (严格)"("Value"=w337) -> ()  [unwired: 2 in, 2 out]
        n214 = call "FGV_VISA_Comm.vi"("Write?"=TRUE, "error in"=w340, "VISA resource name"=w341) -> ()  [unwired: 6 in, 3 out]
      }
      frame "Query_CURRent" {
        # "查询当前输出电流值"
        n215 = call "FGV_VISA_Comm.vi"() -> ("error out"=w354:errorcluster, "VISA resource name out"=w356:refnum<visa-resource-name>)  [unwired: 9 in, 1 out]
        n216 = call <userlib>:"Read CURRent.vi"("error in (no error)"=w354, "等待时间（毫秒）"=u32 50, "Current Tab"=T9."current", "VISA resource name"=w356) -> ("error out"=w353:errorcluster, "Current"=w351:dbl, "VISA resource name out"=w355:refnum<visa-resource-name>)  [unwired: 5 in]
        n217 = property on="Current:" class="DigNum (严格)"("Value"=w351) -> ()  [unwired: 2 in, 2 out]
        n218 = call "FGV_VISA_Comm.vi"("Write?"=TRUE, "error in"=w353, "VISA resource name"=w355) -> ()  [unwired: 6 in, 3 out]
      }
      frame "Query_VOLTage PROTection" {
        # "查询当前输出电压保护阀值"
        n219 = call "FGV_VISA_Comm.vi"() -> ("error out"=w362:errorcluster, "VISA resource name out"=w363:refnum<visa-resource-name>)  [unwired: 9 in, 1 out]
        n220 = call <userlib>:"Read VOLTage PROTection LEVel.vi"("error in (no error)"=w362, "VOLTage Tab"=T8."VOLTage", "VISA resource name"=w363) -> ("error out"=w360:errorcluster, "VOLTage protection level"=w358:dbl, "VISA resource name out"=w361:refnum<visa-resource-name>)  [unwired: 6 in]
        n221 = property on="OVP:" class="DigNum (严格)"("Value"=w358) -> ()  [unwired: 2 in, 2 out]
        n222 = call "FGV_VISA_Comm.vi"("Write?"=TRUE, "error in"=w360, "VISA resource name"=w361) -> ()  [unwired: 6 in, 3 out]
      }
      frame "Query_CURRent PROTection" {
        # "查询当前输出电流保护阀值"
        n223 = call "FGV_VISA_Comm.vi"() -> ("error out"=w369:errorcluster, "VISA resource name out"=w370:refnum<visa-resource-name>)  [unwired: 9 in, 1 out]
        n224 = call <userlib>:"Read CURRent PROTection LEVel.vi"("error in (no error)"=w369, "Current Tab"=T9."current", "VISA resource name"=w370) -> ("error out"=w366:errorcluster, "Current protection level"=w365:dbl, "VISA resource name out"=w367:refnum<visa-resource-name>)  [unwired: 6 in]
        n225 = property on="OCP:" class="DigNum (严格)"("Value"=w365) -> ()  [unwired: 2 in, 2 out]
        n226 = call "FGV_VISA_Comm.vi"("Write?"=TRUE, "error in"=w366, "VISA resource name"=w367) -> ()  [unwired: 6 in, 3 out]
      }
      frame "Query_VOLTage PROTection ENABle" {
        # "查询当前输出电压保护电路是否使能"
        n227 = call "FGV_VISA_Comm.vi"() -> ("error out"=w374:errorcluster, "VISA resource name out"=w375:refnum<visa-resource-name>)  [unwired: 9 in, 1 out]
        n228 = call <userlib>:"Read VOLTage PROTection STATus.vi"("error in (no error)"=w374, "VISA resource name"=w375) -> ("error out"=w373:errorcluster, "VOLTage Protection Status"=w372:bool, "VISA resource name out"=w376:refnum<visa-resource-name>)  [unwired: 6 in, 1 out]
        n229 = property on="OVPEnable" class="Bool (严格)"("Value"=w372) -> ()  [unwired: 2 in, 2 out]
        n230 = call "FGV_VISA_Comm.vi"("Write?"=TRUE, "error in"=w373, "VISA resource name"=w376) -> ()  [unwired: 6 in, 3 out]
      }
      frame "Query_CURRent PROTection ENABle" {
        # "查询当前输出电流保护电路是否使能"
        n231 = call "FGV_VISA_Comm.vi"() -> ("error out"=w381:errorcluster, "VISA resource name out"=w382:refnum<visa-resource-name>)  [unwired: 9 in, 1 out]
        n232 = call <userlib>:"Read CURRent PROTection STATus.vi"("error in (no error)"=w381, "VISA resource name"=w382) -> ("error out"=w379:errorcluster, "Current Protection Status"=w378:bool, "VISA resource name out"=w380:refnum<visa-resource-name>)  [unwired: 6 in, 1 out]
        n233 = property on="OCPEnable" class="Bool (严格)"("Value"=w378) -> ()  [unwired: 2 in, 2 out]
        n234 = call "FGV_VISA_Comm.vi"("Write?"=TRUE, "error in"=w379, "VISA resource name"=w380) -> ()  [unwired: 6 in, 3 out]
      }
      frame "Query_OUTPut" {
        # "查询通道输出状态"
        n235 = call "FGV_VISA_Comm.vi"() -> ("error out"=w387:errorcluster, "VISA resource name out"=w389:refnum<visa-resource-name>)  [unwired: 9 in, 1 out]
        n236 = call <userlib>:"Read OUTPut ENABle.vi"("error in (no error)"=w387, "等待时间（毫秒）"=u32 50, "VISA resource name"=w389) -> ("error out"=w386:errorcluster, "OUTPut Status"=w385:bool, "VISA resource name out"=w388:refnum<visa-resource-name>)  [unwired: 6 in]
        n237 = property on="On/Off" class="Bool (严格)"("Value"=w385) -> ()  [unwired: 2 in, 2 out]
        n238 = call "FGV_VISA_Comm.vi"("Write?"=TRUE, "error in"=w386, "VISA resource name"=w388) -> ()  [unwired: 6 in, 3 out]
      }
      frame "Exit" {
        # "退出"
        n239 = To Variant(anything=FALSE) -> (Variant=w401:variant)
        n240 = Bundle By Name(cluster=cluster{"Instruct":string, "Data":variant} {"Instruct"="", "Data"=variant} ("通知"), "Instruct"="Exit", "Data"=w401) -> (w404:cluster{"Instruct":string, "Data":variant})
        n241 = Send Notification(notification=w404, notifier=w400) -> ()  [unwired: 1 in, 2 out]
        n242 = property on="ExecuteTime(s)" class="DigNum (严格)"() -> ("Value"=w399:dbl)  [unwired: 2 in, 2 out]
        n243 = property on="BufferTime(s)" class="DigNum (严格)"() -> ("Value"=w398:dbl)  [unwired: 2 in, 2 out]
        n244 = property on="Step voltage:" class="DigNum (严格)"() -> ("Value"=w397:dbl)  [unwired: 2 in, 2 out]
        n245 = property on="Max voltage:" class="DigNum (严格)"() -> ("Value"=w396:dbl)  [unwired: 2 in, 2 out]
        n246 = Build Array(w399, w398, w397, w396) -> (w395:dbl[])
        n247 = Flatten To XML(6:w395) -> (2:w394:string)
        n248 = call "Examine Path.vi"("Filename"="MianData.xml") -> ("error out"=w393:errorcluster, "Path"=w392:path)  [unwired: 9 in]
        n249 = call-poly <vilib>:"Write to XML File.vi"("error in (no error)"=w393, "XML Input"=w394, "XML File Path"=w392) -> ()  [unwired: 6 in, 3 out]
      }
    }
  }
  n250 = while {
    tunnel: w27 -> [_]
    stop <- w410 stop-if-true
    n251 = event shown="[4] \"PCAN Config\": 值改变" {
      selector: _ -> [_ _ _ _ _ _ _ _ _ _ _ _ _ _]
      dyn-events: _ -> [_ _ _ _ _ _ _ _ _ _ _ _ _ _]
      timeout: 20 -> [_ _ _ _ _ _ _ _ _ _ _ _ _ _]
      tunnel: [w429 w475 string[] ["Config_Reset"] ("Instruct") string[] ["VISA_Close", "VISA_Config", "VISA_Open", "Config_Off", "Query_OUTPut", "Query_VORTage", "Query_CURRent", "Query_VOLTage PROTection", "Query_CURRent PROTection", "Query_VOLTage PROTection ENABle", "Query_CURRent PROTection ENABle"] ("Instruct") string[] ["PCAN_Close", "PCAN_Config", "PCAN_Open"] ("Instruct") string[] ["Transmit_info"] ("Instruct") string[] ["Config_VOLTage"] ("Instruct") string[] ["Config_CURRent"] ("Instruct") string[] ["Config_VOLTage PROTection"] ("Instruct") string[] ["Config_CURRent PROTection"] ("Instruct") string[] ["Config_VOLTage PROTection ENABle"] ("Instruct") string[] ["Config_CURRent PROTection ENABle"] ("Instruct") _ string[] ["Config_Off", "Config_VOLTage", "VISA_Close", "PCAN_Close", "Exit"] ("Instruct")] -> w412
      tunnel: [w428 _ _ _ _ _ _ _ _ _ _ _ _ variant[] [] ("Data")] -> w411
      tunnel: [_ _ _ _ _ _ _ _ _ _ _ _ _ TRUE] -> w410
      event Timeout {
        n252 = event-data() -> ()  [unwired: 1 in, 3 out]
        n253 = property on="BufferTime(s)" class="DigNum (严格)"() -> ("Value"=w418:dbl)  [unwired: 2 in, 2 out]
        n254 = property on="Max voltage" class="DigNum (严格)"() -> ("Value"=w423:dbl)  [unwired: 2 in, 2 out]
        n255 = property on="On/Off" class="Bool (严格)"() -> ("Value"=w415:bool)  [unwired: 2 in, 2 out]
        n256 = Not Equal To 0?(x=w418) -> (x != 0?=w417:bool)
        n257 = feedback-in #2(w415) -> ()
        n258 = feedback #2(FALSE ("Value")) -> (w426:bool)
        n259 = feedback #3(0.0) -> (w420:dbl)
        n260 = Less Or Equal?(x=w420, y="Max voltage:") -> (x <= y?=w419:bool)
        n261 = Less?(x=w420, y=w423) -> (x < y?=w422:bool)
        n262 = Compound Arithmetic op=AND ("复合运算")(w415, w422, w419, w417) -> (w424:bool)
        n263 = case shown="假" w424 {
          tunnel: [w435 w454] -> w429
          tunnel: [w436 w453] -> w416
          tunnel: w420 -> [w430 w451]
          tunnel: [_ w452] -> w428
          tunnel: w426 -> [_ w450]
          tunnel: w419 -> [w433 _]
          tunnel: w415 -> [w432 _]
          frame False {
            n264 = Not(x=w433) -> (.not. x?=w431:bool)
            n265 = And(x=w432, y=w431) -> (x .and. y?=w434:bool)
            n266 = case shown="真" w434 {
              tunnel: [_ string[] ["Save record", "Config_Off", "Config_VOLTage", "Query_OUTPut"] ("Instruct")] -> w435
              tunnel: w431 -> [w438 _]
              tunnel: w430 -> [w437 _]
              frame False {
                n267 = case shown="真" w438 {
                  tunnel: w437 -> [_ w440]
                  frame False {
                  }
                  frame True {
                    n268 = Increment(x=w440) -> (x+1=w439:dbl)
                    n269 = property on="Max voltage:" class="DigNum (严格)"("Value"=w439) -> ()  [unwired: 2 in, 2 out]
                  }
                }
              }
              frame True {
                w441 = T10."Enabled" ("禁用")
                n270 = property on="Voltage:" class="DigNum (严格)"("DisabledEnum"=w441) -> ()  [unwired: 2 in, 2 out]
                n271 = property on="PCAN Config" class="Bool"("DisabledEnum"=w441) -> ()  [unwired: 2 in, 2 out]
                n272 = property on="OVP:" class="DigNum (严格)"("DisabledEnum"=w441) -> ()  [unwired: 2 in, 2 out]
                n273 = property on="OVPEnable" class="Bool (严格)"("DisabledEnum"=w441) -> ()  [unwired: 2 in, 2 out]
                n274 = property on="RS232 Config" class="Bool"("DisabledEnum"=w441) -> ()  [unwired: 2 in, 2 out]
                n275 = property on="Current:" class="DigNum (严格)"("DisabledEnum"=w441) -> ()  [unwired: 2 in, 2 out]
                n276 = property on="Transmit info" class="Bool"("DisabledEnum"=w441) -> ()  [unwired: 2 in, 2 out]
                n277 = property on="OCP:" class="DigNum (严格)"("DisabledEnum"=w441) -> ()  [unwired: 2 in, 2 out]
                n278 = property on="OCPEnable" class="Bool (严格)"("DisabledEnum"=w441) -> ()  [unwired: 2 in, 2 out]
              }
            }
            n279 = property on="Voltage:" class="DigNum (严格)"() -> ("Value"=w436:dbl)  [unwired: 2 in, 2 out]
          }
          frame True {
            n280 = Not(x=w450) -> (.not. x?=w445:bool)
            n281 = Add(x="ExecuteTime(s)", y="BufferTime(s)") -> (x+y=w448:dbl)
            n282 = call "已用时间"("Time Target (s)"=w448, "Reset"=w445) -> ("Elapsed Time (s)"=w446:dbl, "Time has Elapsed"=w455:bool)  [unwired: 10 in, 6 out]
            n283 = Add(x="ExecuteTime(s)", y=1.0) -> (x+y=w443:dbl)
            n284 = case shown="假" w455 {
              tunnel: [w461 string[] ["Config_VOLTage1", "Config_On"] ("Instruct")] -> w454
              tunnel: [w464 w466] -> w453
              tunnel: w451 -> [w464 w469]
              tunnel: [_ w467] -> w452
              tunnel: w446 -> [w463 _]
              tunnel: w445 -> [w459 _]
              tunnel: "ExecuteTime(s)" -> [w457 _]
              tunnel: w443 -> [w456 _]
              frame False {
                n285 = Greater?(x=w463, y=w456) -> (0:w460:bool)
                n286 = Or(x=w460, y=w459) -> (x .or. y?=w458:bool)
                n287 = call "已用时间2"("Time Target (s)"=w457, "Reset"=w458) -> ("Time has Elapsed"=w462:bool)  [unwired: 10 in, 7 out]
                n288 = case shown="真" w462 {
                  tunnel: [_ string[] ["record", "Config_Off"] ("Instruct")] -> w461
                  frame False {
                  }
                  frame True {
                  }
                }
              }
              frame True {
                n289 = Add(x=w469, y="Step voltage:") -> (x+y=w466:dbl)
                n290 = To Variant(anything=w466) -> (Variant=w468:variant)
                n291 = Build Array(w468) -> (w467:variant[])
              }
            }
          }
        }
        n292 = feedback-in #3(w416) -> ()
        n293 = property on="At voltage" class="DigNum (严格)"("Value"=w416) -> ()  [unwired: 2 in, 2 out]
      }
      event "On/Off": Value Change {
        n294 = event-data() -> ("NewVal"=w474:bool)  [unwired: 1 in, 5 out]
        n295 = Select(t=string[] ["Config_VOLTage", "Config_CURRent", "Config_On"] ("Instruct"), s=w474, f=string[] ["Config_Off", "Save record", "Config_VOLTage", "Config_CURRent"] ("Instruct")) -> (s? t:f=w475:string[])
        n296 = case shown="真" w474 {
          tunnel: ["Await the opportune moment" "Begin testing"] -> w473
          tunnel: [T10."Enabled" ("禁用") T10."Disabled and Grayed Out" ("禁用")] -> w472
          frame False {
          }
          frame True {
            n297 = property on="List record" class="MCListbox (严格)"("ItemNames"=string[][] [] ("项名")) -> ()  [unwired: 2 in, 2 out]
          }
        }
        n298 = property on="Voltage:" class="DigNum (严格)"("DisabledEnum"=w472) -> ()  [unwired: 2 in, 2 out]
        n299 = property on="PCAN Config" class="Bool"("DisabledEnum"=w472) -> ()  [unwired: 2 in, 2 out]
        n300 = property on="OVP:" class="DigNum (严格)"("DisabledEnum"=w472) -> ()  [unwired: 2 in, 2 out]
        n301 = property on="OVPEnable" class="Bool (严格)"("DisabledEnum"=w472) -> ()  [unwired: 2 in, 2 out]
        n302 = property on="Status:" class="Str"("Value"=w473) -> ()  [unwired: 2 in, 2 out]
        n303 = property on="RS232 Config" class="Bool"("DisabledEnum"=w472) -> ()  [unwired: 2 in, 2 out]
        n304 = property on="Current:" class="DigNum (严格)"("DisabledEnum"=w472) -> ()  [unwired: 2 in, 2 out]
        n305 = property on="Transmit info" class="Bool"("DisabledEnum"=w472) -> ()  [unwired: 2 in, 2 out]
        n306 = property on="OCP:" class="DigNum (严格)"("DisabledEnum"=w472) -> ()  [unwired: 2 in, 2 out]
        n307 = property on="OCPEnable" class="Bool (严格)"("DisabledEnum"=w472) -> ()  [unwired: 2 in, 2 out]
      }
      event "Reset": Value Change {
        n308 = event-data() -> ()  [unwired: 1 in, 6 out]
        n309 = property on="Status:" class="Str"("Value"="Reset") -> ()  [unwired: 2 in, 2 out]
      }
      event "RS232 Config": Value Change {
        n310 = event-data() -> ()  [unwired: 1 in, 6 out]
        n311 = property on="Status:" class="Str"("Value"="RS232 Config") -> ()  [unwired: 2 in, 2 out]
      }
      event "PCAN Config": Value Change {
        n312 = event-data() -> ()  [unwired: 1 in, 6 out]
        n313 = property on="Status:" class="Str"("Value"="PCAN Config") -> ()  [unwired: 2 in, 2 out]
      }
      event "Transmit info": Value Change {
        n314 = event-data() -> ()  [unwired: 1 in, 6 out]
        n315 = property on="Status:" class="Str"("Value"="Transmit info") -> ()  [unwired: 2 in, 2 out]
      }
      event "Voltage:": Value Change {
        n316 = event-data() -> ()  [unwired: 1 in, 6 out]
      }
      event "Current:": Value Change {
        n317 = event-data() -> ()  [unwired: 1 in, 6 out]
      }
      event "OVP:": Value Change {
        n318 = event-data() -> ()  [unwired: 1 in, 6 out]
      }
      event "OCP:": Value Change {
        n319 = event-data() -> ()  [unwired: 1 in, 6 out]
      }
      event "OVPEnable": Value Change {
        n320 = event-data() -> ()  [unwired: 1 in, 6 out]
      }
      event "OCPEnable": Value Change {
        n321 = event-data() -> ()  [unwired: 1 in, 6 out]
      }
      event "Receive": Mouse Down {
        n322 = event-data() -> ("CtlRef"=w500:refnum<vi>, "Coords"=w499:T11)  [unwired: 1 in, 6 out]
        n323 = invoke class="MCListbox (严格)" method="Point To Row Column"(reference=w500, "Point"=w499) -> ("CellPosition"=w498:T12)  [unwired: 5 in, 6 out]
        n324 = Unbundle By Name(w498) -> ("Row"=w497:i32)
        n325 = property on="Receive" class="MCListbox (严格)"("Value"=w497) -> ()  [unwired: 2 in, 2 out]
      }
      event Panel Close? {
        n326 = event-data() -> ()  [unwired: 1 in, 4 out]
        n327 = property on="Status:" class="Str"("Value"="Exit") -> ()  [unwired: 2 in, 2 out]
        n328 = event-data("Discard?"=TRUE ("放弃？")) -> ()  [unwired: 1 in, 1 out]
      }
    }
    n329 = Format Date/Time String(time format string (%c)="%Y/%m/%d %H:%M:%S" ("时间格式字符串(%c)")) -> (date/time string=→"Time:":string)  [unwired: 2 in]
    n330 = call "Queue.vi"("State"=QueueState."In", "Data"=w411, "Instruct"=w412) -> ()  [unwired: 6 in, 3 out]
    "Company:" <- "Hinge-teck" ("Company:")
  }
  n331 = while {
    tunnel: w20 -> [w507]
    tunnel: w18 -> [w521]
    shift-right: [w512] -> _
    shift-left: "" ("Instruct") -> [w518]
    shift-right: [w511] -> _
    shift-left: FALSE -> [w513]
    tunnel: w19 -> [w508]
    tunnel: [w508] -> w8
    tunnel: [w507] -> w16
    stop <- w510 stop-if-true
    w506 = 10 ("超时毫秒(-1)")
    # "PCAN Write"
    n332 = Wait on Notification(notifier=w521, timeout in ms (-1)=w506, error in (no error)=w507) -> (notification=w520:cluster{"Instruct":string, "Data":variant})  [unwired: 1 in, 3 out]
    n333 = Unbundle By Name(w520) -> ("Instruct"=w519:string, "Data"=w516:variant)
    n334 = Variant To Data(type=FALSE, Variant=w516) -> (data=w514:bool, error out=w509:errorcluster)  [unwired: 1 in]
    n335 = Empty String/Path?(string/path=w519) -> (empty?=w517:bool)
    n336 = Select(t=w518, s=w517, f=w519) -> (s? t:f=w512:string)
    n337 = call <vilib>:"Clear Errors.vi"("error in (no error)"=w509) -> ()  [unwired: 5 in, 2 out]
    n338 = Select(t=w513, s=w517, f=w514) -> (s? t:f=w511:bool)
    n339 = case shown="\"Start\"" w512 {
      tunnel: w511 -> [_ _ _]
      tunnel: [_ _ TRUE] -> w510
      tunnel: w508 -> [_ w526 _]
      tunnel: w506 -> [_ w522 _]
      frame "假", Default {
      }
      frame "Start" {
        n340 = Dequeue Element(queue=w526, timeout in ms (-1)=w522) -> (element=w525:cluster{"instruct":string, "data":variant})  [unwired: 1 in, 3 out]
        n341 = Unbundle By Name(w525) -> ("instruct"=w524:string, "data"=w523:variant)
        n342 = case shown="\"PCAN_Write\"" w524 {
          tunnel: w523 -> [_ w533]
          frame "假", Default {
          }
          frame "PCAN_Write" {
            n343 = Tick Count (ms)() -> (millisecond timer value=w528:u32)
            n344 = feedback-in #4(w528) -> ()
            n345 = feedback #4() -> (w527:u32)  [unwired: 1 in]
            n346 = Subtract(x=w528, y=w527) -> (x-y=→"x-y":u32)
            n347 = Variant To Data(type=T13 [] ("MessageBuffer"), Variant=w533) -> (data=w531:T13)  [unwired: 1 in, 1 out]
            n348 = call "FGV_PCAN_Config.vi"() -> ("Channel out"=w530:T1)  [unwired: 8 in, 3 out]
            n349 = for {
              tunnel: w531 -> [w534] mode=indexing
              tunnel: w530 -> [w535]
              tunnel: [w534] -> _ mode=indexing
              n350 = call <userlib>:"CAN Write.vi"("Channel"=w535, "MessageBuffer"=w534) -> ()  [unwired: 2 out]
            }
          }
        }
      }
      frame "Exit" {
      }
    }
  }
  n351 = while {
    tunnel: w19 -> [w557]
    tunnel: w6 -> [w556]
    tunnel: w20 -> [w541]
    tunnel: w18 -> [w553]
    shift-right: [w543] -> _
    shift-left: "" ("Instruct") -> [w546]
    shift-right: [w545] -> _
    shift-left: FALSE -> [w544]
    tunnel: [w541] -> w17
    stop <- w542 stop-if-true
    n352 = property on="LastError" class="Str"() -> ("Value"=w538:string)  [unwired: 2 in, 2 out]
    n353 = Wait on Notification(notifier=w553, timeout in ms (-1)=10 ("超时毫秒(-1)"), error in (no error)=w541) -> (notification=w554:cluster{"Instruct":string, "Data":variant})  [unwired: 1 in, 3 out]
    n354 = Unbundle By Name(w554) -> ("Instruct"=w547:string, "Data"=w548:variant)
    n355 = Variant To Data(type=FALSE, Variant=w548) -> (data=w550:bool, error out=w549:errorcluster)  [unwired: 1 in]
    n356 = call "Connect error.vi"("LastError"=w538, "PCAN Read error"="PCAN Read error", "source"="source") -> ("LastError out"=→"LastError":string)  [unwired: 8 in]
    n357 = Empty String/Path?(string/path=w547) -> (empty?=w552:bool)
    n358 = call <vilib>:"Clear Errors.vi"("error in (no error)"=w549) -> ()  [unwired: 5 in, 2 out]
    n359 = Select(t=w546, s=w552, f=w547) -> (s? t:f=w543:string)
    n360 = Select(t=w544, s=w552, f=w550) -> (s? t:f=w545:bool)
    n361 = case shown="\"Start\"" w543 {
      tunnel: w557 -> [_ w563 _]
      tunnel: w556 -> [_ w562 _]
      tunnel: [_ _ TRUE] -> w542
      frame "假", Default {
      }
      frame "Start" {
        n362 = call "Conformity.vi"() -> ("整合后"=w560:T14, "时间段"=w559:u16[])  [unwired: 10 in]
        n363 = call "Timing.vi"("数组"=w559) -> ("当前"=w561:u16, "到"=w558:bool)  [unwired: 8 in, 1 out]
        n364 = case shown="真" w558 {
          tunnel: w563 -> [_ w565]
          tunnel: w562 -> [_ w564]
          tunnel: w561 -> [_ w567]
          tunnel: w560 -> [_ w566]
          frame False {
          }
          frame True {
            n365 = for {
              tunnel: w566 -> [w574] mode=indexing
              tunnel: w567 -> [w572]
              tunnel: w565 -> [w569]
              tunnel: w564 -> [w568]
              n366 = Unbundle By Name(w574) -> ("Time"=w573:u16, "MessageBuffer"=w570:T13)
              n367 = Equal?(x=w572, y=w573) -> (x = y?=w571:bool)
              n368 = case shown="真" w571 {
                tunnel: w570 -> [_ w580]
                tunnel: w569 -> [_ w579]
                tunnel: w568 -> [_ w578]
                frame False {
                }
                frame True {
                  n369 = To Variant(anything=w580) -> (Variant=w575:variant)
                  n370 = Bundle By Name(cluster=cluster{"instruct":string, "data":variant} {"instruct"="PCAN_Write", "data"=variant}, "data"=w575) -> (w577:cluster{"instruct":string, "data":variant})
                  n371 = Enqueue Element(queue=w579, element=w577, error in (no error)=w578) -> ()  [unwired: 1 in, 3 out]
                }
              }
            }
          }
        }
      }
      frame "Exit" {
      }
    }
  }
  n372 = Release Queue(queue=w8) -> ()  [unwired: 2 in, 3 out]
  n373 = property on="Status" class="Bool (严格)" props=["Value"]() -> ()  [unwired: 2 in, 3 out]
  n374 = call "Queue.vi"("State"=QueueState."Close", "error in"=w22) -> ()  [unwired: 7 in, 3 out]
  n375 = Merge Errors(w14, w16, w17) -> (w13:errorcluster)
  n376 = control-ref of="本VI"() -> (w2:refnum<vi>)
  n377 = Release Notifier(notifier=w12, error in (no error)=w13) -> (error out=w1:errorcluster)  [unwired: 1 in, 2 out]
  n378 = invoke class="VI" method="FP.Close"(reference=w2, error in=w1) -> ()  [unwired: 1 in, 3 out]
